vi "TriggeredFrequencySweep.vi"() -> ()   [LabVIEW 2018]
uses:
  <vilib>/express/express analysis/Spectral/Block/exnSpectralBlock spectral measurements RMS poly.vi
  <vilib>/express/express analysis/Spectral/Block/exnSpectralBlock spectral measurements RMS DDT.vi
  <vilib>/express/express analysis/Spectral/XNode/ExpressSpectralMeasurementsBlockNode.xnode
panel:
  out "Saving Data":bool
  out "Filename Out":path
  in  "Filename":path=path "C:/Users/joud/Documents/Joud Tests_Data_VI/Frequency Sweep/FRF Test Fs40Hz.lvm"
  in  "Enable":bool=TRUE
  in  "Reset":bool
  out "data 3":dynamicdata(graph) caption="data"
  in  "device name":tag="cDAQ6Mod1"
  in  "stop (T)":bool=TRUE
  in  "timeout (s)":dbl=10.0 format="%0.2f"
  in  "number of samples":i32=3060000
  in  "rate":dbl=1651.0
  out "data 2":dynamicdata(graph) caption="data"
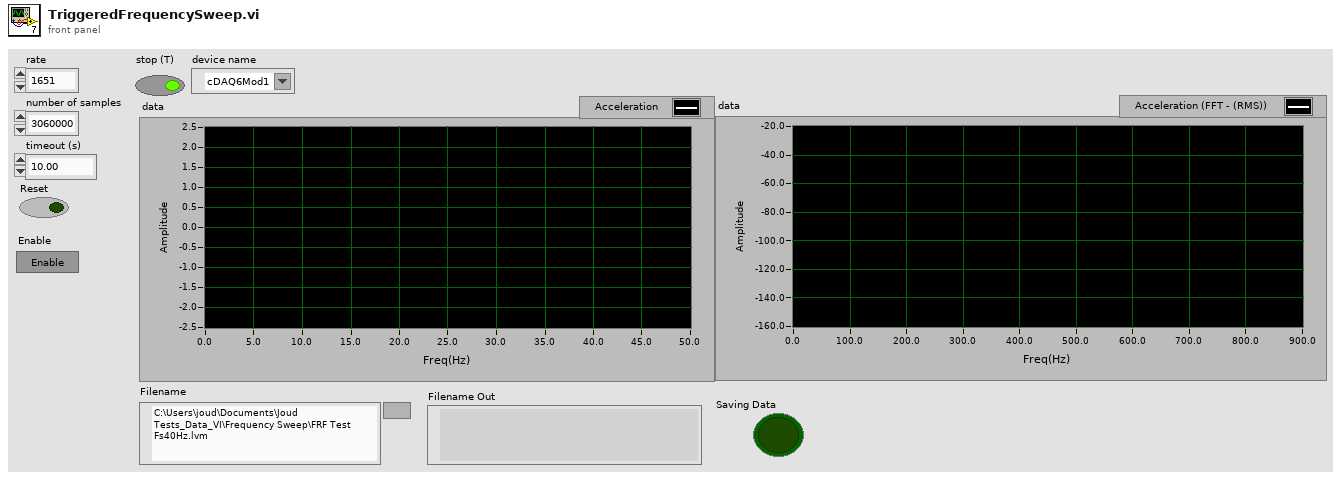
[diagram p1: front panel]
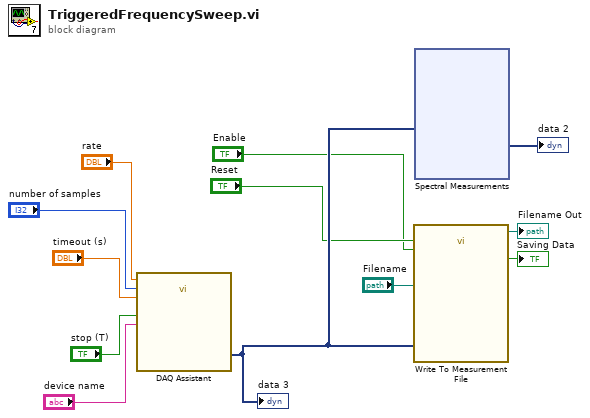
[diagram p0: block diagram]
diagram:
  n1 = call "DAQ Assistant"("rate"="rate", "number of samples"="number of samples", "timeout (s)"="timeout (s)", "stop (T)"="stop (T)", "device name"="device name") -> ("data"=w6:dynamicdata)  [unwired: 12 in, 2 out]
  "data 3" <- w6
  n2 = call "Write To Measurement File"("Signals"=w6, "Reset"="Reset", "Enable"="Enable", "Filename"="Filename") -> ("Filename Out"=→"Filename Out":path, "Saving Data"=→"Saving Data":bool)  [unwired: 13 in, 1 out]
  n3 = xnode "Spectral Measurements"("Signals"=w6) -> ("FFT - (RMS)"=→"data 2":dynamicdata)  [unwired: 1 in, 2 out]
